vi "check_tables (SubVI).vi"(6 "bool in":bool, 9 "numeric buffer in":dbl, 10 "temperature array in":dbl[](array[numeric]), 11 "Data in":T1) -> (2 "temperature array out":dbl[](array[numeric]), 3 "Data out":T1)   [LabVIEW 2015]
uses:
  data_typedef.ctl
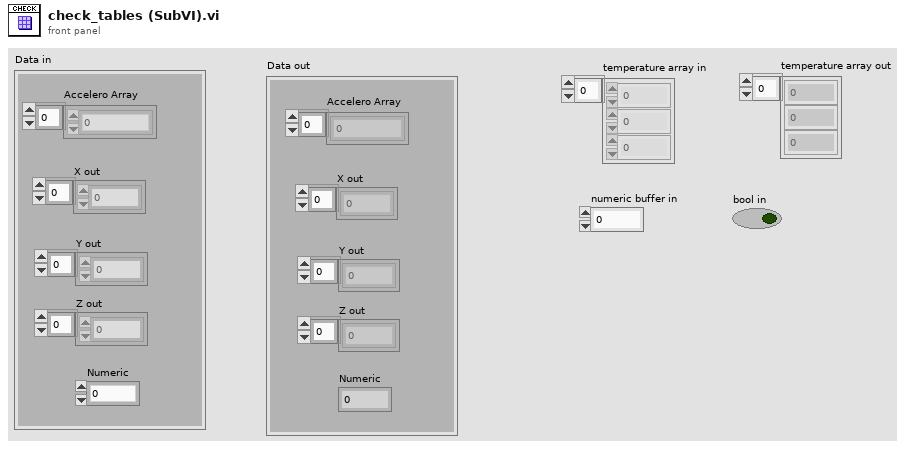
[diagram p1: front panel]
types:
  T1 = typedef "data_typedef.ctl" = cluster{"Accelero Array":dbl[], "Z out":dbl[], "Y out":dbl[], "X out":dbl[], "Numeric":i32}
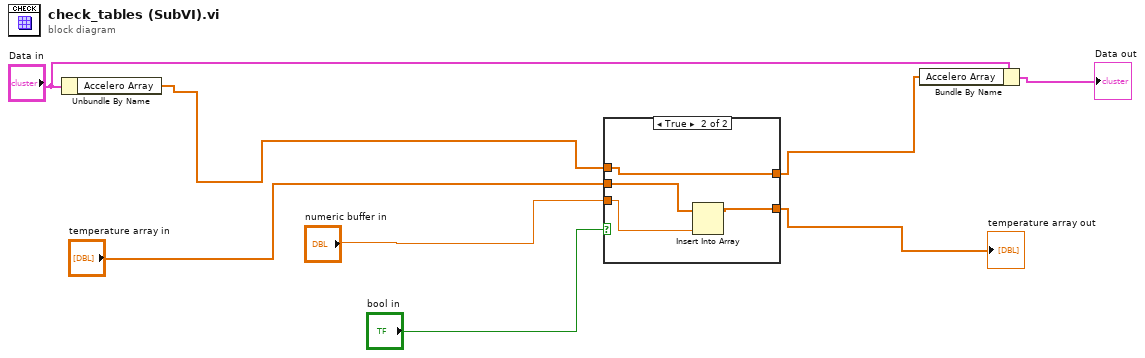
[diagram p0: block diagram]
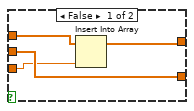
[diagram p2: hidden frame]
diagram:
  n1 = Unbundle By Name("Data in") -> ("Accelero Array"=w4:dbl[])
  n2 = case shown="True" "bool in" {
    tunnel: "numeric buffer in" -> [w10 w15]
    tunnel: w4 -> [w11 w16]
    tunnel: "temperature array in" -> [w12 w14]
    tunnel: [w12 w13] -> w5
    tunnel: [w9 w16] -> w2
    frame False {
      n3 = Insert Into Array(array=w11, new element=w10) -> (w9:dbl[])  [unwired: 1 in]
    }
    frame True {
      n4 = Insert Into Array(array=w14, new element=w15) -> (w13:dbl[])  [unwired: 1 in]
    }
  }
  "temperature array out" <- w5
  n5 = Bundle By Name(cluster="Data in", "Accelero Array"=w2) -> (→"Data out":T1)
